vi "AB_Log_Close.vi"(8 "error in (no error)":errorcluster) -> (0 "error out":errorcluster)   [LabVIEW 2020]
uses:
  <vilib>/AppBuilder/logging/AB_Log_File_Action.ctl
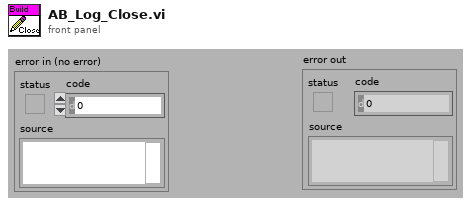
[diagram p1: front panel]
types:
  T1 = typedef "AB_Log_File_Action.ctl" = enum16{"write", "open", "close"}
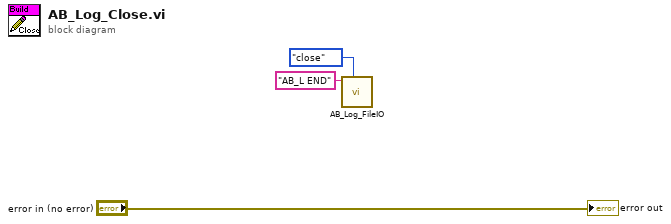
[diagram p0: block diagram]
diagram:
  n1 = call <vilib>:"AB_Log_FileIO.vi"("fileAction"=AB_Log_File_Action."close", "newSection"="AB_L END") -> ()  [unwired: 9 in, 1 out]
  "error out" <- "error in (no error)"
